vi "DistanceBetweenPointsOnEachScanLine.vi"(6 "Search Lines":T2[](array[typedef]) {"Edge Info"."Distance (Real-World)" format="%.2f"; "Edge Info"."Location (Real-World)"."Y" format="%.2g"; "Edge Info"."Location (Real-World)"."X" format="%.2f"; "Edge Info"."Noise" format="%.2f"; "Edge Info"."Location (Pixel)"."Y" format="%.2g"; "Edge Info"."Location (Pixel)"."X" format="%.2f"; "Edge Info"."Strength" format="%.2f"; "Edge Info"."Distance (Pixel)" format="%.2f"}, 7 "Refnum in":T3, 8 "error in (no error)":errorcluster, 9 "Last Edges":T1[](array[typedef]) {"Distance (Real-World)" format="%.2f"; "Location (Real-World)"."Y" format="%.2g"; "Location (Real-World)"."X" format="%.2f"; "Noise" format="%.2f"; "Location (Pixel)"."Y" format="%.2g"; "Location (Pixel)"."X" format="%.2f"; "Strength" format="%.2f"; "Distance (Pixel)" format="%.2f"}, 10 "First Edges":T1[](array[typedef]) {"Distance (Real-World)" format="%.2f"; "Location (Real-World)"."Y" format="%.2g"; "Location (Real-World)"."X" format="%.2f"; "Noise" format="%.2f"; "Location (Pixel)"."Y" format="%.2g"; "Location (Pixel)"."X" format="%.2f"; "Strength" format="%.2f"; "Distance (Pixel)" format="%.2f"}, 11 "Refnum in":T3) -> (0 "error out":errorcluster, 1 "NumberOfIternations":i32, 2 "Array":sgl[](array[numeric]), 3 "Numeric":i32)   [LabVIEW 2015]
uses:
  <vilib>/vision/Image Controls.llb/IMAQ Image.ctl
  <vilib>/vision/Measure.llb/Search Line.ctl
  <vilib>/vision/Measure.llb/Edge New.ctl
  <vilib>/vision/NI_Vision_Development_Module.lvlib
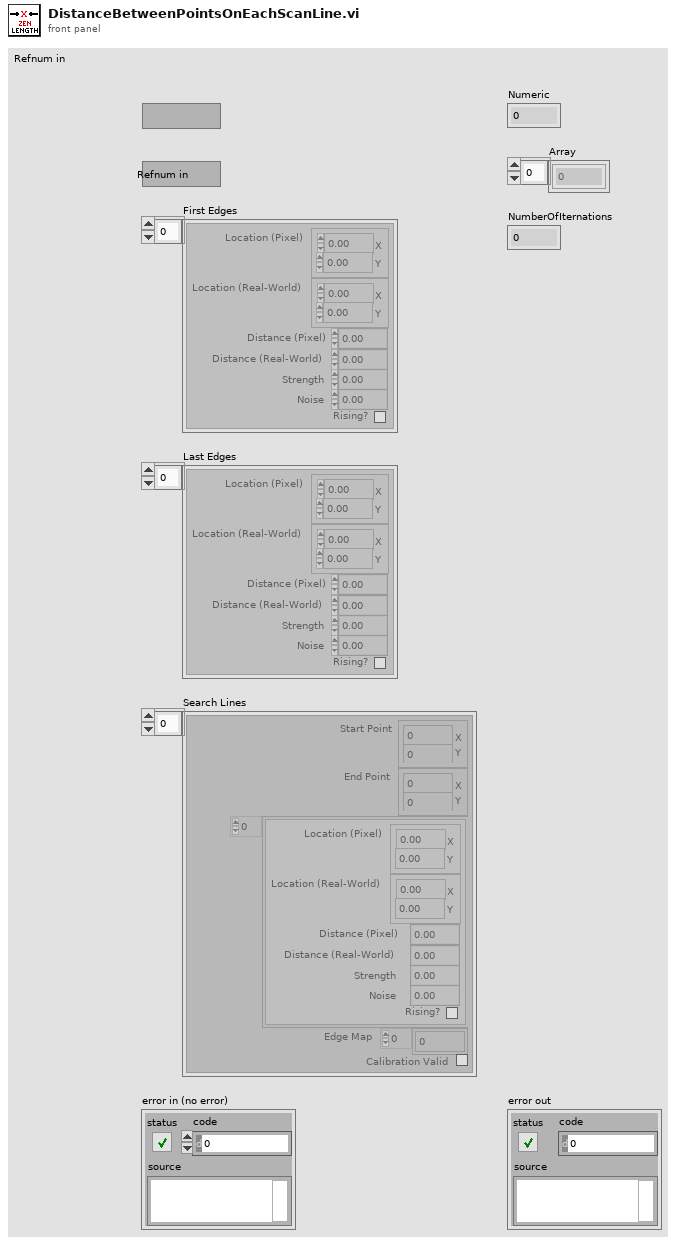
[diagram p1: front panel]
types:
  T1 = typedef "Edge New.ctl" = cluster{"Location (Pixel)":cluster{"X":sgl, "Y":sgl}, "Location (Real-World)":cluster{"X":sgl, "Y":sgl}, "Distance (Pixel)":dbl, "Distance (Real-World)":dbl, "Strength":dbl, "Noise":dbl, "Rising?":bool}
  T2 = typedef "Search Line.ctl" = cluster{"Start Point":cluster{"X":sgl, "Y":sgl}, "End Point":cluster{"X":sgl, "Y":sgl}, "Edge Info":T1[], "Edge Map":dbl[], "Calibration Valid":bool}
  T3 = typedef "IMAQ Image.ctl" = refnum<image>
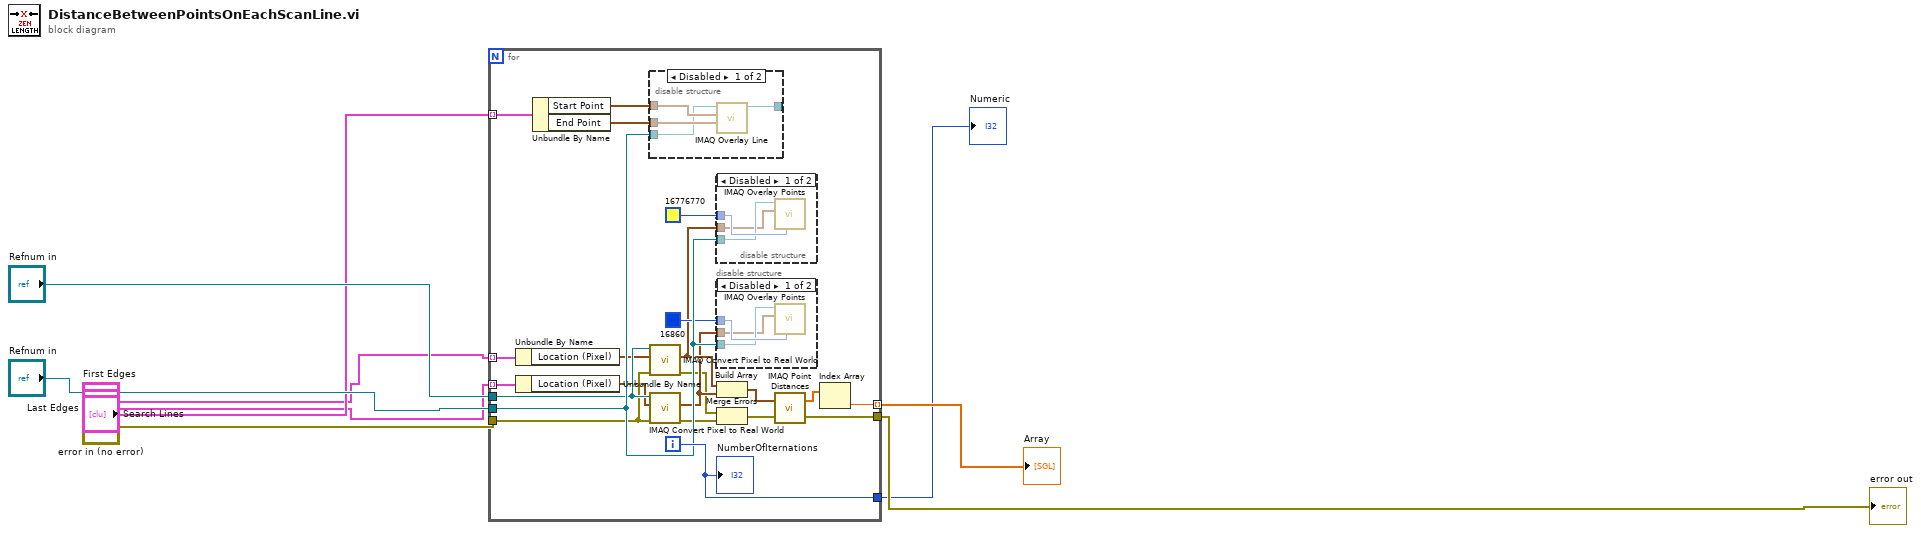
[diagram p0: block diagram]
diagram:
  n1 = for {
    tunnel: "Refnum in" -> [w24]
    tunnel: "First Edges" -> [w31] mode=indexing
    tunnel: "Last Edges" -> [w30] mode=indexing
    tunnel: "Search Lines" -> [w29] mode=indexing
    tunnel: [w25] -> w2 mode=indexing
    tunnel: [w26] -> w1
    tunnel: "Refnum in" -> [w23]
    tunnel: "error in (no error)" -> [w22]
    tunnel: [w21] -> w4
    i -> [w26]
    n2 = Unbundle By Name(w31) -> ("Location (Pixel)"=w15:cluster{"X":sgl, "Y":sgl})
    n3 = Unbundle By Name(w30) -> ("Location (Pixel)"=w14:cluster{"X":sgl, "Y":sgl})
    n4 = Unbundle By Name(w29) -> ("Start Point"=w28:cluster{"X":sgl, "Y":sgl}, "End Point"=w27:cluster{"X":sgl, "Y":sgl})
    n5 = disable-structure shown="Disabled" {
      disable-tunnel: w28 -> [w41 _]
      disable-tunnel: w27 -> [w40 _]
      disable-tunnel: w24 -> [w39 _]
      disable-tunnel: [w38 _] -> _
      frame Disabled {
        n6 = call "IMAQ Overlay Line"("End Point"=w40, "Start Point"=w41, "Image"=w39) -> ("Image Out"=w38:T3)  [unwired: 7 in, 1 out]
      }
      frame Enabled {
      }
    }
    n7 = call "IMAQ Convert Pixel to Real World"("error in (no error)"=w22, "Pixel Coordinates"=w15, "Calibrated Image"=w23) -> ("error out"=w12:errorcluster, "Real World Coordinates"=w16:cluster{"X":sgl, "Y":sgl})  [unwired: 3 in, 4 out]
    n8 = call "IMAQ Convert Pixel to Real World"("error in (no error)"=w22, "Pixel Coordinates"=w14, "Calibrated Image"=w23) -> ("error out"=w11:errorcluster, "Real World Coordinates"=w13:cluster{"X":sgl, "Y":sgl})  [unwired: 3 in, 4 out]
    n9 = disable-structure shown="Disabled" {
      disable-tunnel: u32 16776770 ("Color") -> [w37 _]
      disable-tunnel: w24 -> [w36 _]
      disable-tunnel: w16 -> [w35 _]
      frame Disabled {
        n10 = call "IMAQ Overlay Points"("Color"=w37, "Point"=w35, "Image"=w36) -> ()  [unwired: 7 in, 2 out]
      }
      frame Enabled {
      }
    }
    n11 = disable-structure shown="Disabled" {
      disable-tunnel: u32 16860 ("Color") -> [w34 _]
      disable-tunnel: w24 -> [w33 _]
      disable-tunnel: w13 -> [w32 _]
      frame Disabled {
        n12 = call "IMAQ Overlay Points"("Color"=w34, "Point"=w32, "Image"=w33) -> ()  [unwired: 7 in, 2 out]
      }
      frame Enabled {
      }
    }
    n13 = Build Array(w16, w13) -> (w20:cluster{"X":sgl, "Y":sgl}[])
    n14 = Merge Errors(w12, w11) -> (w10:errorcluster)
    n15 = call "IMAQ Point Distances"("Points"=w20, "error in (no error)"=w10) -> ("Distances"=w19:sgl[], "error out"=w21:errorcluster)  [unwired: 3 in]
    n16 = Index Array(array=w19) -> (element=w25:sgl)  [unwired: 1 in]
    "NumberOfIternations" <- w26
  }
  "error out" <- w4
  "Array" <- w2
  "Numeric" <- w1
